vi "SwissSPAD Live_Update SS2 Gate Definition.vi"(8 "error in (no error)":errorcluster, 10 "Gate Configuration Definition":T1, 11 "SS2 DAQ Parameters Refnum":refnum<vi>) -> (0 "error out":errorcluster, 1 "Reversed Shift":bool, 2 "SS2 DAQ Parameters":T3 {"Sync Period" min=0.0 max=4.294967295; "# Sets" min=1})   [LabVIEW 2021]
uses:
  SwissSPAD Live_SS2 DAQ Parameters 3.ctl
  SwissSPAD Live_SS2 Gate Definition.ctl
  SwissSPAD Live_SS2 Gate Configuration.ctl
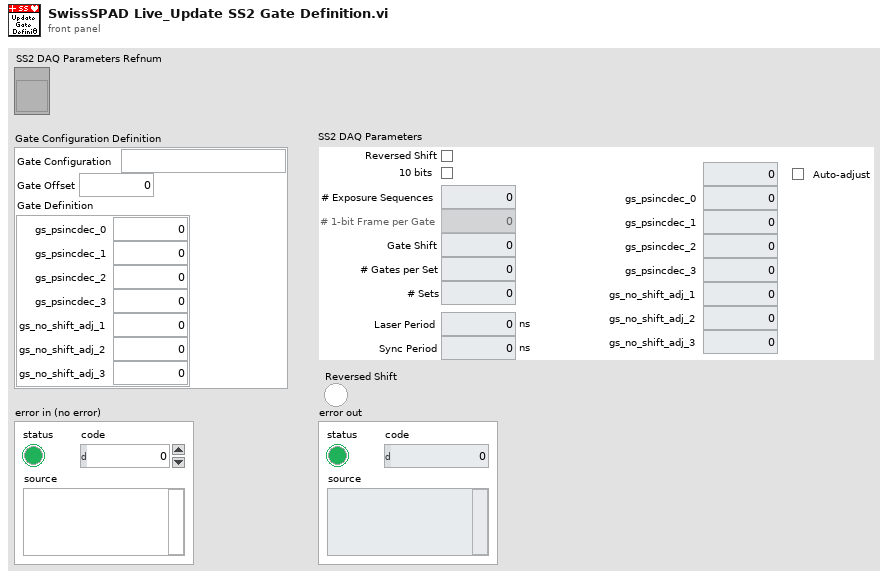
[diagram p1: front panel]
types:
  T1 = typedef "SwissSPAD Live_SS2 Gate Configuration.ctl" = cluster{"Gate Configuration":string, "Gate Offset":u32, "Gate Definition":T2}
  T2 = typedef "SwissSPAD Live_SS2 Gate Definition.ctl" = cluster{"gs_psincdec_0":u32, "gs_psincdec_1":u32, "gs_psincdec_2":u32, "gs_psincdec_3":u32, "gs_no_shift_adj_1":u32, "gs_no_shift_adj_2":u32, "gs_no_shift_adj_3":u32}
  T3 = typedef "SwissSPAD Live_SS2 DAQ Parameters 3.ctl" = cluster{"10 bits":bool, "# Exposure Sequences":u32, "# 1-bit Frame per Gate":u32, "Gate Shift":u32, "# Gates per Set":u32, "# Sets":u32, "Laser Period":dbl[unit], "Sync Period":dbl[unit], "Gate Offset":u32, "Auto-adjust Gate Offset":bool, "Gate Definition":T2, "Reversed Shift":bool}
  T4 = typedef "SwissSPAD Lve_SS2 DAQ Parameters 3.ctl" = cluster{"10 bits":bool, "# Exposure Sequences":u32, "# 1-bit Frame per Gate":u32, "Gate Shift":u32, "# Gates per Set":u32, "# Sets":u32, "Laser Period":dbl[unit], "Sync Period":dbl[unit], "Gate Offset":u32, "Auto-adjust Gate Offset":bool, "Gate Definition":T2, "Reversed Shift":bool}
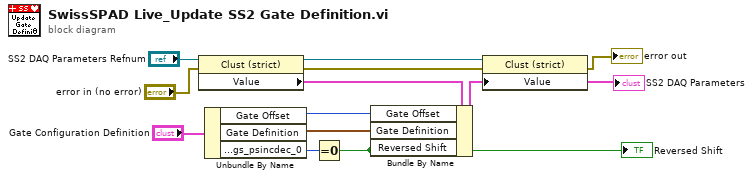
[diagram p0: block diagram]
diagram:
  n1 = property class="Clust (strict)"(reference="SS2 DAQ Parameters Refnum", error in="error in (no error)") -> (reference out=w11:refnum<vi>, error out=w10:errorcluster, "Value"=w7:T4)
  n2 = Unbundle By Name("Gate Configuration Definition") -> ("Gate Offset"=w5:u32, "Gate Definition"=w4:T2, "Gate Definition.gs_psincdec_0"=w2:u32)
  n3 = Equal To 0?(x=w2) -> (x = 0?=w1:bool)
  "Reversed Shift" <- w1
  n4 = Bundle By Name(cluster=w7, "Gate Offset"=w5, "Gate Definition"=w4, "Reversed Shift"=w1) -> (w6:T4)
  "SS2 DAQ Parameters" <- w6
  n5 = property class="Clust (strict)"(reference=w11, error in=w10, "Value"=w6) -> (error out=→"error out":errorcluster)  [unwired: 1 out]
